vi "STICK-SetDAC.vi"(4 "error in (no error)":errorcluster, 6 "IDA 0 [V]":dbl min=0.0 max=2.0, 7 "VISA resource name":refnum<visa-resource-name>) -> (0 "error out":errorcluster, 3 "VISA resource name out":refnum<visa-resource-name>)   [LabVIEW 2014]
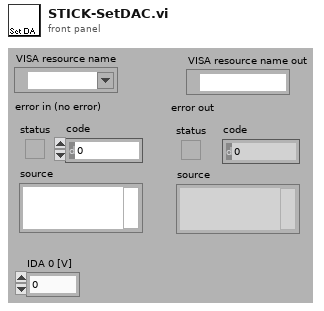
[diagram p1: front panel]
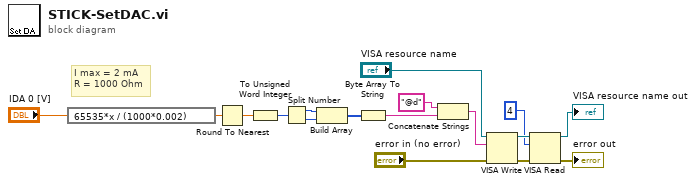
[diagram p0: block diagram]
diagram:
  # "I max = 2 mA\nR = 1000 Ohm"
  n1 = expression code="65535*x / (1000*0.002)"("IDA 0 [V]") -> (w6:dbl)
  n2 = Round To Nearest(number=w6) -> (nearest integer value=w5:dbl)
  n3 = To Unsigned Word Integer(number=w5) -> (unsigned 16bit integer=w3:u16)
  n4 = Split Number(x=w3) -> (hi(x)=w17:u8, lo(x)=w16:u8)
  n5 = Build Array(w17, w16) -> (w15:u8[])
  n6 = Byte Array To String(unsigned byte array=w15) -> (string=w11:string)
  n7 = Concatenate Strings("@d", w11) -> (w10:string)
  n8 = VISA Write(VISA resource name="VISA resource name", write buffer=w10, error in (no error)="error in (no error)") -> (VISA resource name out=w9:refnum<visa-resource-name>, error out=w8:errorcluster)  [unwired: 1 out]
  n9 = VISA Read(VISA resource name=w9, byte count=u32 4, error in (no error)=w8) -> (VISA resource name out=→"VISA resource name out":refnum<visa-resource-name>, error out=→"error out":errorcluster)  [unwired: 2 out]
